vi "TCP Read xTP Reply.vi"(8 "error in (no error)":errorcluster, 10 "Num Retries":i32=5, 11 "buffered tcp connection":refnum<k5>) -> (0 "error out":errorcluster, 1 "reply code":i32, 2 "reply string":string, 3 "buffered tcp connection out":refnum<k5>)   [LabVIEW 2020, in "NI_FTP.lvlib"]
doc: "Reads lines from a connection created with TCP Buffered Open.\nThe data is assumed to be in the response format used by FTP, SMTP, etc.\nWhen a line that begins with three digits followed by a space is encountered, all the lines (including this last one) are returned in \"reply string\". The number is returned in \"reply code\"."
uses:
  <vilib>/FTP/NI_FTP.lvlib
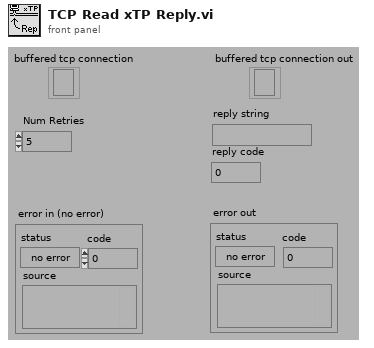
[diagram p1: front panel]
types:
  T1 = enum16{"Standard", "Buffered", "CRLF", "Immediate"}
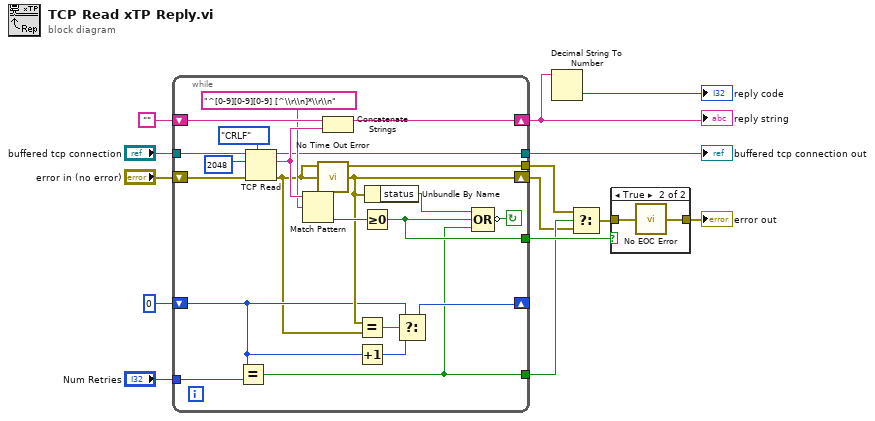
[diagram p0: block diagram]
diagram:
  n1 = while {
    tunnel: [w25] -> w9
    tunnel: [w26] -> w11
    tunnel: "buffered tcp connection" -> [w31]
    shift-left: "error in (no error)" -> [w32]
    shift-right: [w22] -> w3
    shift-left: "" -> [w29]
    shift-right: [w28] -> w13
    shift-right: [w19] -> _
    shift-left: 0 -> [w18]
    tunnel: "Num Retries" -> [w17]
    tunnel: [w16] -> w4
    tunnel: [w15] -> w2
    stop <- w34 continue-if-true
    n2 = Equal?(x=w18, y=w17) -> (x = y?=w16:bool)
    n3 = TCP Read(connection ID=w31, bytes to read=2048, error in (no error)=w32, 7:T1."CRLF" ("mode (standard)")) -> (connection ID out=w26:refnum<k5>, data out=w30:string, error out=w15:errorcluster)  [unwired: 1 out]
    n4 = Match Pattern(string=w30, regular expression="^[0-9][0-9][0-9] [^\\r\\n]*\\r\\n") -> (offset past match=w33:i32)  [unwired: 4 out]
    n5 = call <vilib>:"No Time Out Error.vi"("error in (no error)"=w15) -> ("error out"=w22:errorcluster)  [unwired: 14 out]
    n6 = Concatenate Strings(w29, w30) -> (w28:string)
    n7 = Equal?(x=w22, y=w15) -> (x = y?=w21:bool)
    n8 = Increment(x=w18) -> (x+1=w20:i32)
    n9 = Greater Or Equal To 0?(x=w33) -> (x >= 0?=w25:bool)
    n10 = Unbundle By Name(w22) -> ("status"=w35:bool)
    n11 = Select(t=w18, s=w21, f=w20) -> (s? t:f=w19:i32)
    n12 = Compound Arithmetic op=OR(w35, w25, w16) -> (invert w34:bool)
  }
  "buffered tcp connection out" <- w11
  "reply string" <- w13
  n13 = Decimal String To Number(string=w13) -> (number=→"reply code":i32)  [unwired: 3 out]
  n14 = Select(t=w2, s=w4, f=w3) -> (s? t:f=w5:errorcluster)
  n15 = case shown="True" w9 {
    tunnel: w5 -> [w36 w38]
    tunnel: [w36 w37] -> w6
    frame False {
    }
    frame True {
      n16 = call <vilib>:"No EOC Error.vi"("error in (no error)"=w38) -> ("error out"=w37:errorcluster)  [unwired: 4 out]
    }
  }
  "error out" <- w6
